vi "UT_001_TOML to LV.vi"() -> ()   [LabVIEW 2017]
uses:
  b63e0b88-7ba7-4dee-a43e-fc5dcdf3e80e.vi
  7dc6aa98-3bd4-4305-a38f-b45c177b78e8.vi
  c5341fb9-8734-4d16-865c-83784ba59dbe.vi
  9b204452-4378-4217-8ce8-edfe2d471006.vi
  04455632-4ea7-4004-ad0e-dcc5f65a6605.vi
  88135e47-21b0-4fd1-85e0-e7ee9c587d2f.vi
  lib/TOML to LabVIEW.vi
  <vilib>/addons/_JKI Toolkits/Caraya/classes/Assert/Assert Not Error.vi
  <vilib>/addons/_JKI Toolkits/Caraya/classes/Assert/Assert True.vi
  <vilib>/addons/_JKI Toolkits/Caraya/classes/Assert/Assert Error.vi
  <vilib>/addons/_JKI Toolkits/Caraya/classes/Test/Test.lvclass
  <vilib>/addons/_JKI Toolkits/Caraya/classes/Assert/Assert.lvclass
  lib/TOML.lvlib
panel:
  out "error out":errorcluster
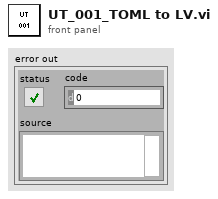
[diagram p1: front panel]
types:
  T1 = cluster{"error":cluster{"sttus":bool, "code":i32, "source":string}}
  T2 = typedef "TOML.lvlib/TOML Value.ctl" = cluster{"type":enum16{"Table", "Array", "String", "Integer", "Float", "Boolean", "Offset Date-Time", "Local Date-Time", "Local Date", "Local Time"}, "value":variant}
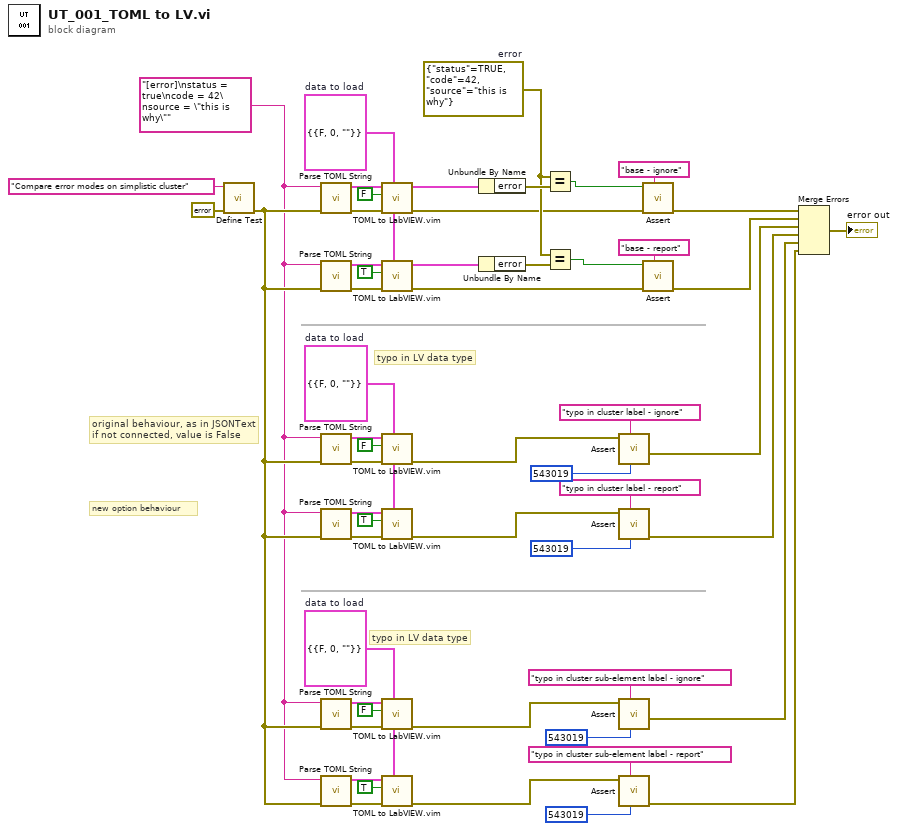
[diagram p0: block diagram]
diagram:
  w14 = T1 {"error"={"sttus"=FALSE, "code"=0, "source"=""}}  # data to load
  w6 = cluster{"errr":errorcluster} {"errr"={"status"=FALSE, "code"=0, "source"=""}}  # data to load
  w25 = cluster{"error":errorcluster} {"error"={"status"=FALSE, "code"=0, "source"=""}}  # data to load
  w39 = errorcluster {"status"=TRUE, "code"=42, "source"="this is why"}  # error
  w32 = "[error]\nstatus = true\ncode = 42\nsource = \"this is why\"" ("String")
  # "new option behaviour"
  # "original behaviour, as in JSONText\nif not connected, value is False"
  # "typo in LV data type"
  # "typo in LV data type"
  n1 = call <vilib>:"Define Test.vi"("error in (no error)"=errorcluster {"status"=FALSE, "code"=0, "source"=""}, "Label (VI Title)"="Compare error modes on simplistic cluster") -> ("error out"=w33:errorcluster)  [unwired: 9 in]
  n2 = call "Parse TOML String.vi"("error in (no error)"=w33, "String"=w32) -> ("error out"=w28:errorcluster, "Value"=w29:T2)  [unwired: 8 in]
  n3 = call "Parse TOML String.vi"("error in (no error)"=w33, "String"=w32) -> ("error out"=w23:errorcluster, "Value"=w26:T2)  [unwired: 8 in]
  n4 = call "Parse TOML String.vi"("error in (no error)"=w33, "String"=w32) -> ("error out"=w4:errorcluster, "Value"=w2:T2)  [unwired: 8 in]
  n5 = call "Parse TOML String.vi"("error in (no error)"=w33, "String"=w32) -> ("error out"=w9:errorcluster, "Value"=w5:T2)  [unwired: 8 in]
  n6 = call "Parse TOML String.vi"("error in (no error)"=w33, "String"=w32) -> ("error out"=w16:errorcluster, "Value"=w18:T2)  [unwired: 8 in]
  n7 = call "Parse TOML String.vi"("error in (no error)"=w33, "String"=w32) -> ("error out"=w11:errorcluster, "Value"=w13:T2)  [unwired: 8 in]
  n8 = call "TOML to LabVIEW.vim"("datatype"=w25, "error in (no error)"=w28, "Error if missing element"=FALSE, "Value"=w29) -> ("error out"=w22:errorcluster, "LV Data"=w27:cluster{"error":errorcluster})  [unwired: 5 in, 1 out]
  n9 = call "TOML to LabVIEW.vim"("datatype"=w25, "error in (no error)"=w23, "Error if missing element"=TRUE, "Value"=w26) -> ("error out"=w21:errorcluster, "LV Data"=w20:cluster{"error":errorcluster})  [unwired: 5 in, 1 out]
  n10 = call "TOML to LabVIEW.vim"("error in (no error)"=w4, "Error if missing element"=FALSE, "Value"=w2) -> ("error out"=w3:errorcluster)  [unwired: 6 in, 2 out]
  n11 = call "TOML to LabVIEW.vim"("datatype"=w6, "error in (no error)"=w9, "Error if missing element"=TRUE, "Value"=w5) -> ("error out"=w7:errorcluster)  [unwired: 5 in, 2 out]
  n12 = call "TOML to LabVIEW.vim"("datatype"=w14, "error in (no error)"=w16, "Error if missing element"=FALSE, "Value"=w18) -> ("error out"=w15:errorcluster)  [unwired: 5 in, 2 out]
  n13 = call "TOML to LabVIEW.vim"("datatype"=w14, "error in (no error)"=w11, "Error if missing element"=TRUE, "Value"=w13) -> ("error out"=w10:errorcluster)  [unwired: 5 in, 2 out]
  n14 = Unbundle By Name(w27) -> ("error"=w49:errorcluster)
  n15 = Unbundle By Name(w20) -> ("error"=w42:errorcluster)
  n16 = Equal?(x=w39, y=w49) -> (x = y?=w51:bool)
  n17 = Equal?(x=w39, y=w42) -> (x = y?=w41:bool)
  n18 = call-poly <vilib>:"Assert.vi"("error code (1)"=543019, "Label"="typo in cluster label - ignore" ("Label (VI Title)"), "Not Error?"=w3) -> ("error out"=w47:errorcluster)  [unwired: 8 in]
  n19 = call-poly <vilib>:"Assert.vi"("error code (1)"=543019, "Label"="typo in cluster label - report" ("Label (VI Title)"), "Error?"=w7) -> ("error out"=w30:errorcluster)  [unwired: 8 in]
  n20 = call-poly <vilib>:"Assert.vi"("error code (1)"=543019, "Label"="typo in cluster sub-element label - ignore" ("Label (VI Title)"), "Not Error?"=w15) -> ("error out"=w45:errorcluster)  [unwired: 8 in]
  n21 = call-poly <vilib>:"Assert.vi"("error code (1)"=543019, "Label"="typo in cluster sub-element label - report" ("Label (VI Title)"), "Error?"=w10) -> ("error out"=w31:errorcluster)  [unwired: 8 in]
  n22 = call-poly <vilib>:"Assert.vi"("Label"="base - ignore" ("Label (VI Title)"), "error in (no error)"=w22, "True?"=w51) -> ("error out"=w54:errorcluster)  [unwired: 8 in]
  n23 = call-poly <vilib>:"Assert.vi"("Label"="base - report" ("Label (VI Title)"), "error in (no error)"=w21, "True?"=w41) -> ("error out"=w38:errorcluster)  [unwired: 8 in]
  n24 = Merge Errors(w54, w38, w47, w30, w45, w31) -> (→"error out":errorcluster)
